vi "IDS_RILIS_V2.vi"() -> ()   [LabVIEW 2015]
uses:
  Case_Selector.ctl
  <vilib>/Utility/file.llb/Read Delimited Spreadsheet (DBL).vi
panel:
  in  "Manual Start":bool
  out "Integral2":dbl
  out "Integral1":dbl
  out "IDS Spectrum":cluster{"all rows":dbl[], "all rows":dbl[]}(graph)
  out "Run Number":dbl
  out "Path":string
  out "IDS_Status.sh - ERROR":string
  out "IDS_Sort.sh - ERROR":string
  out "IDS Data Taking":bool
  out "IDS Sorting":bool
  out "loop counter":i32
  out "RILIS ERROR":bool
  out "IDS ERROR":bool
  out "RILIS Ready":bool
  out "HFS Scan Graph 2":cluster{"Y":dbl[], "Y":dbl[]}[](graph)
  out "Integral":dbl[](array[numeric]) format="%#.2f"
  out "?":string
  out "IDS Ready":bool
  out "IDS_Start.sh - ERROR":string
  out "?":string
  out "Wavenumber Stdev":dbl
  out "Proton Pulses in SC":dbl format="%#_10g"
  out "Full Name":string
  out "created path":path
  in  "stop":bool
  out "Proton Pulse":bool
  out "Super Cycle":bool
  out "protons per pulse":dbl
  out "StepNumber":i32
  out "Wavenumber":dbl format="%#_11g"
  out "Measurement time stamp":timestamp
  out "Laser Power":dbl format="%#_11g"
  out "Integrated current":dbl
  in  "File Base":string
  # "Measurement time stamp"
  # "Output"
  # "RILIS"
  # "Separator"
  # "IDS"
  # "Results"
  # "Last update: 22 May 2022 \nAuthors: Ralf Erik Rossel, Razvan Lica, Rob Harding"
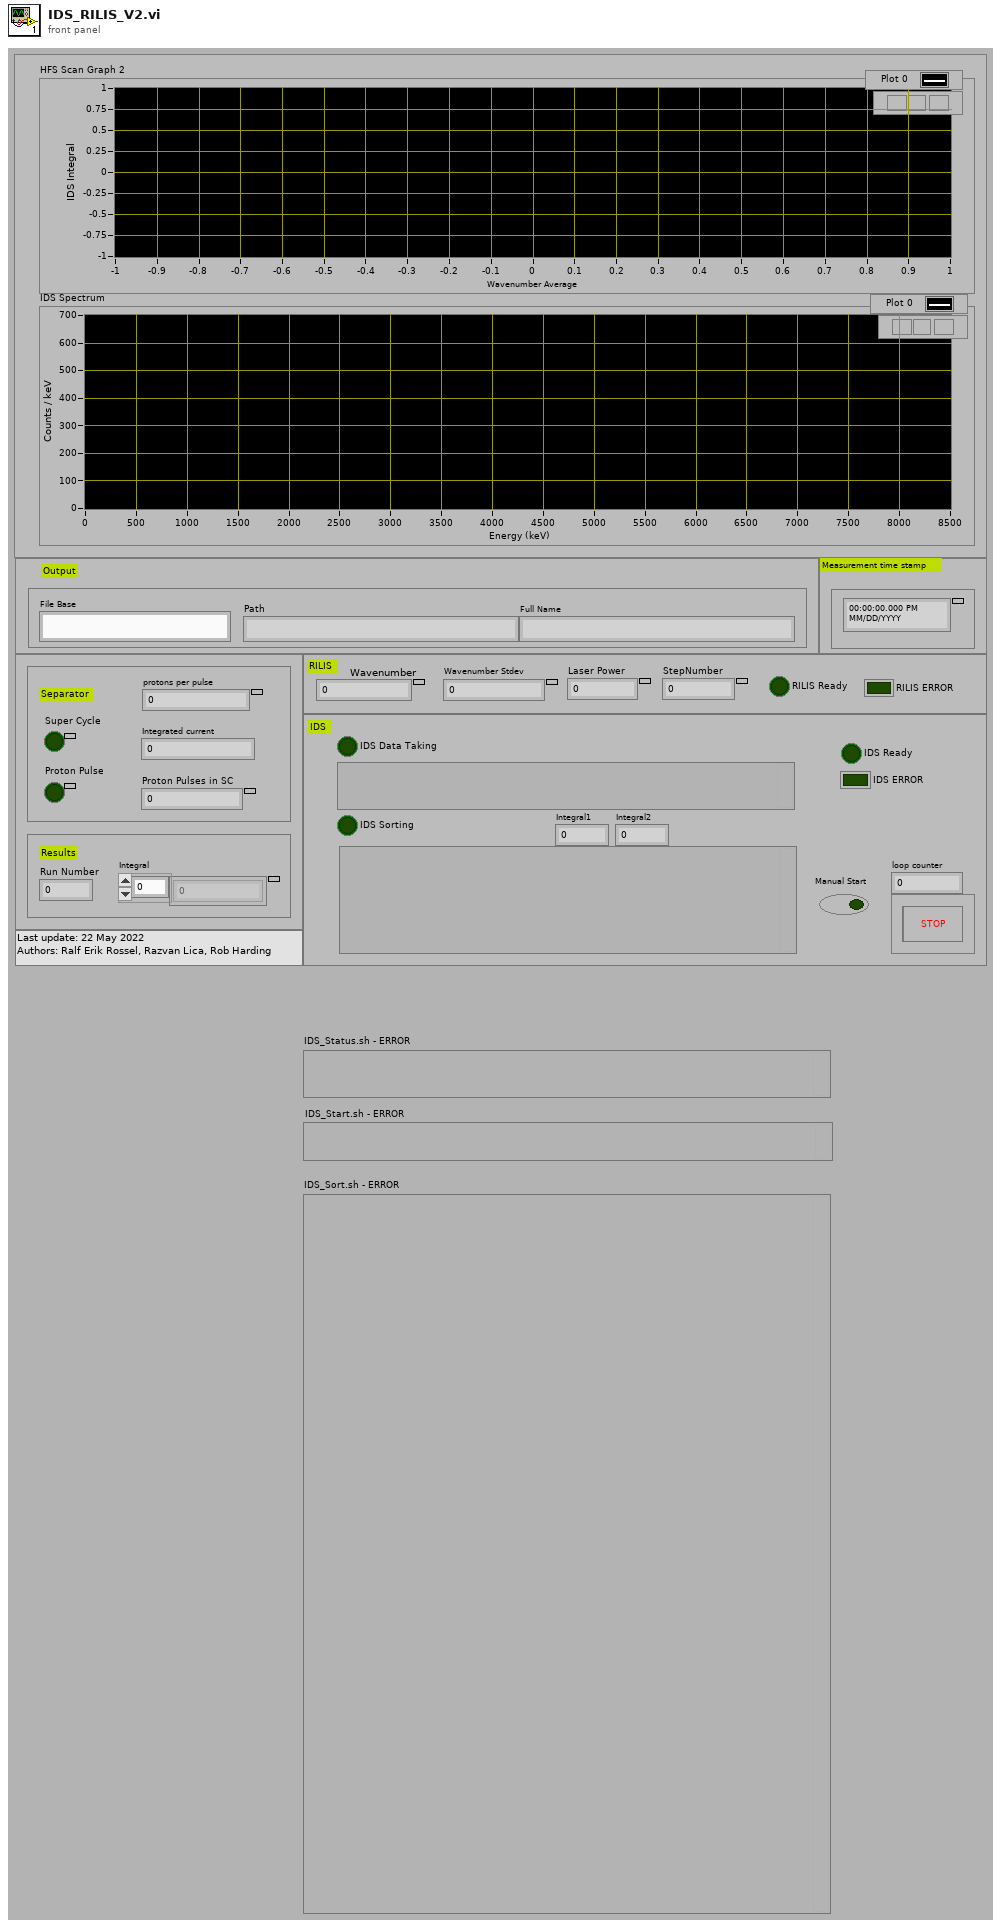
[diagram p1: front panel]
types:
  T1 = typedef "Case_Selector.ctl" = enum16{"RILIS Init", "RILIS On", "RILIS AQN", "RILIS SORT"}
  T2 = enum16{"open", "replace", "create", "open or create", "replace or create", "replace or create with confirmation"}
  T3 = enum16{"Read", "Write", "ReadWrite", "BufferedRead", "BufferedReadWrite"}
  T4 = cluster{"[0]":dbl, "[1]":dbl, "[2]":dbl, "[3]":dbl, "[4]":dbl, "[5]":dbl, "[6]":dbl, "[7]":dbl, "[8]":dbl}
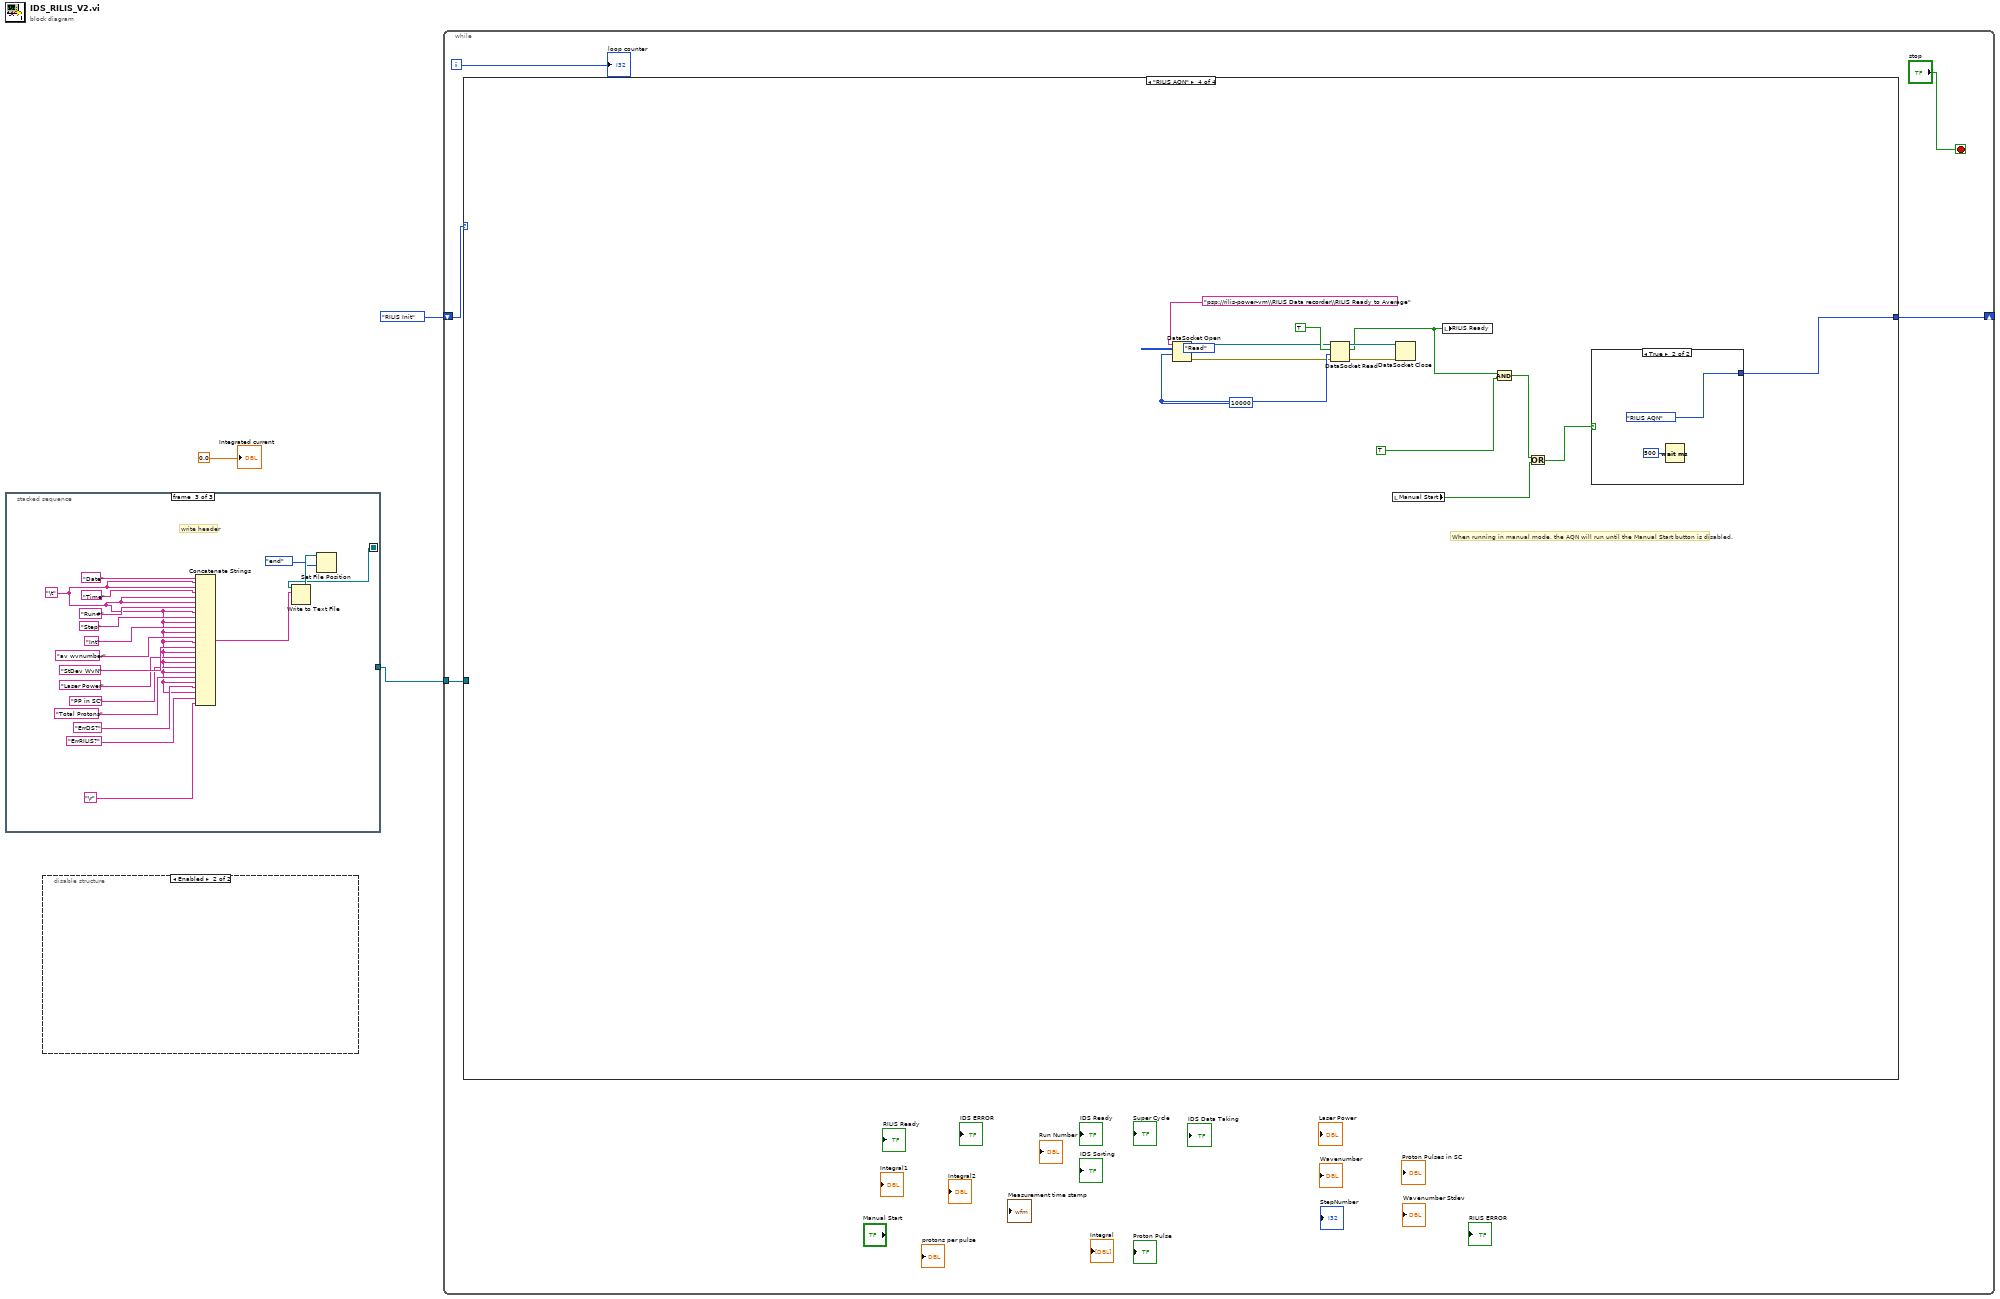
[diagram p0: block diagram]
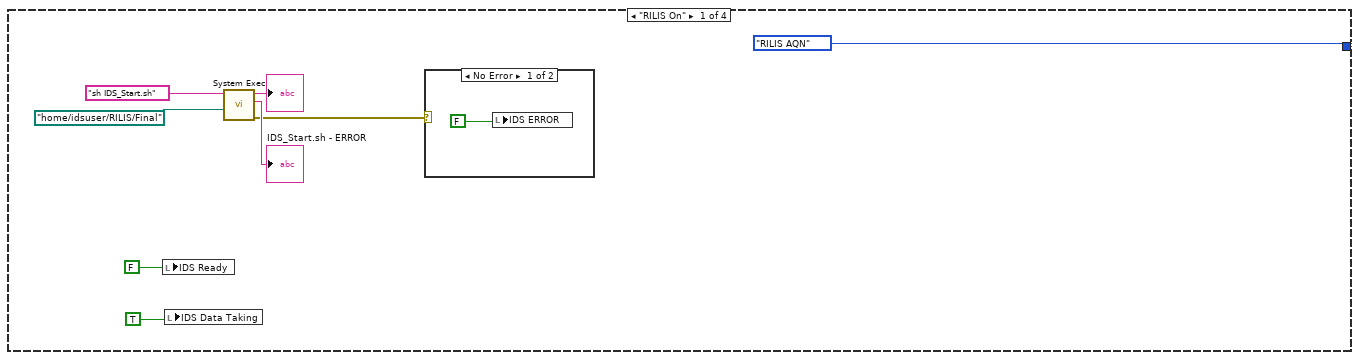
[diagram p2: hidden frame]
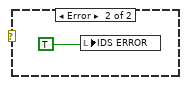
[diagram p3: hidden frame]
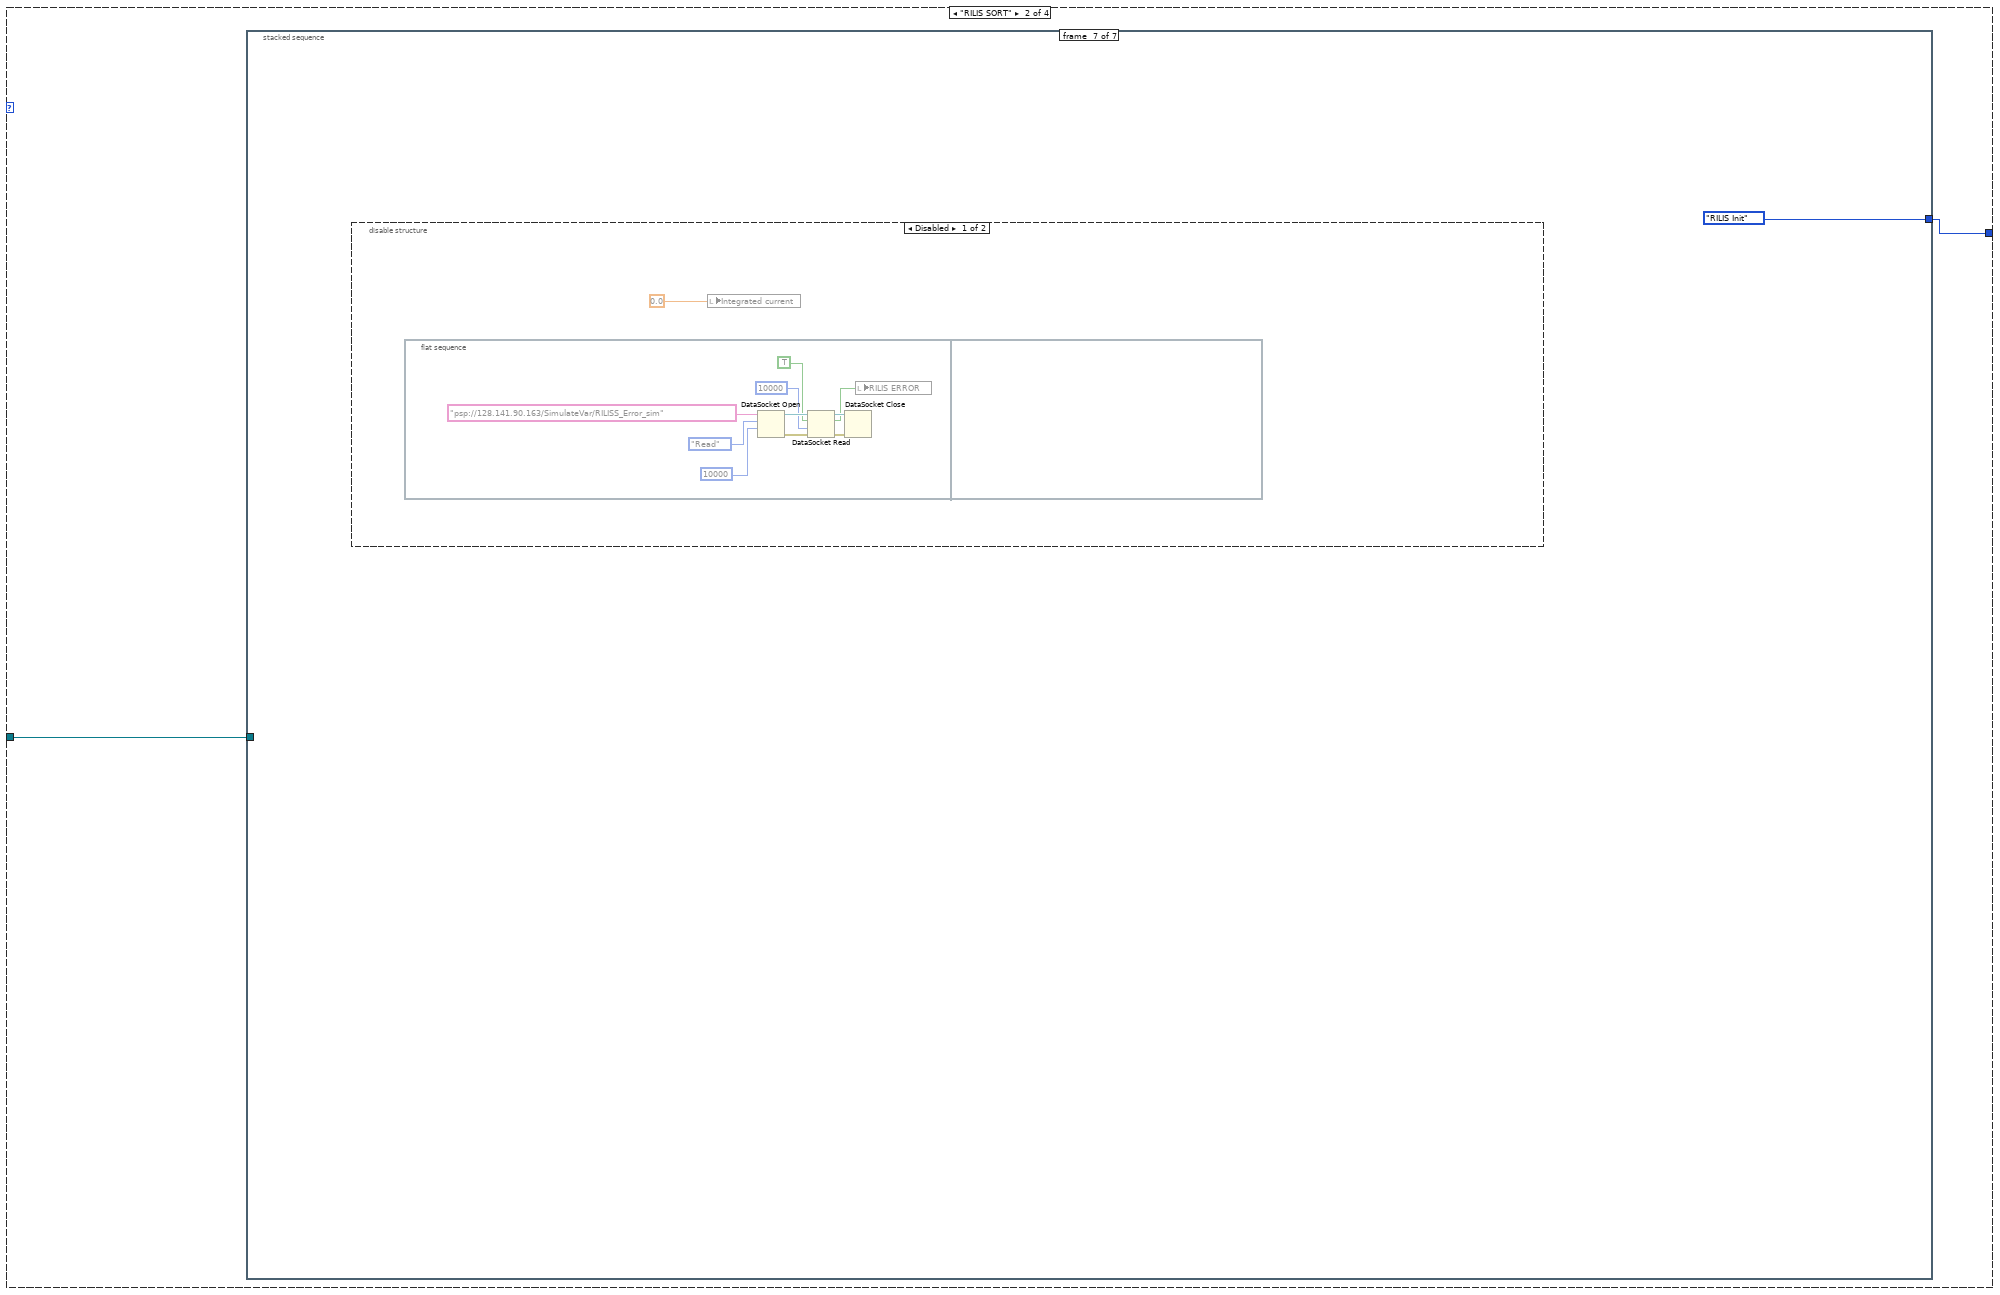
[diagram p4: hidden frame]
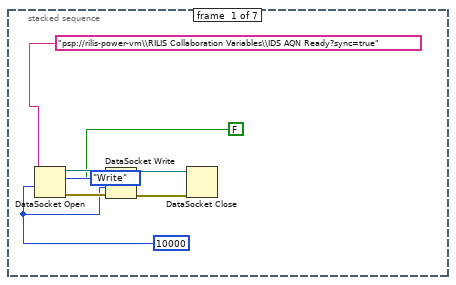
[diagram p5: hidden frame]
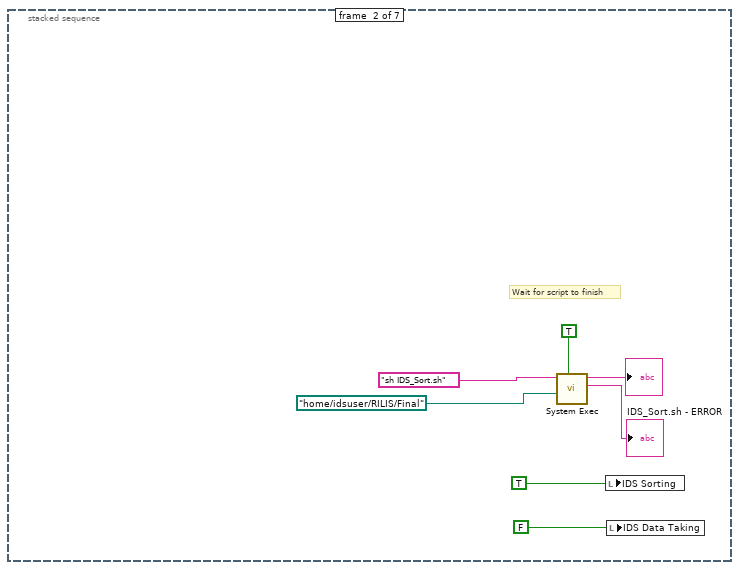
[diagram p6: hidden frame]
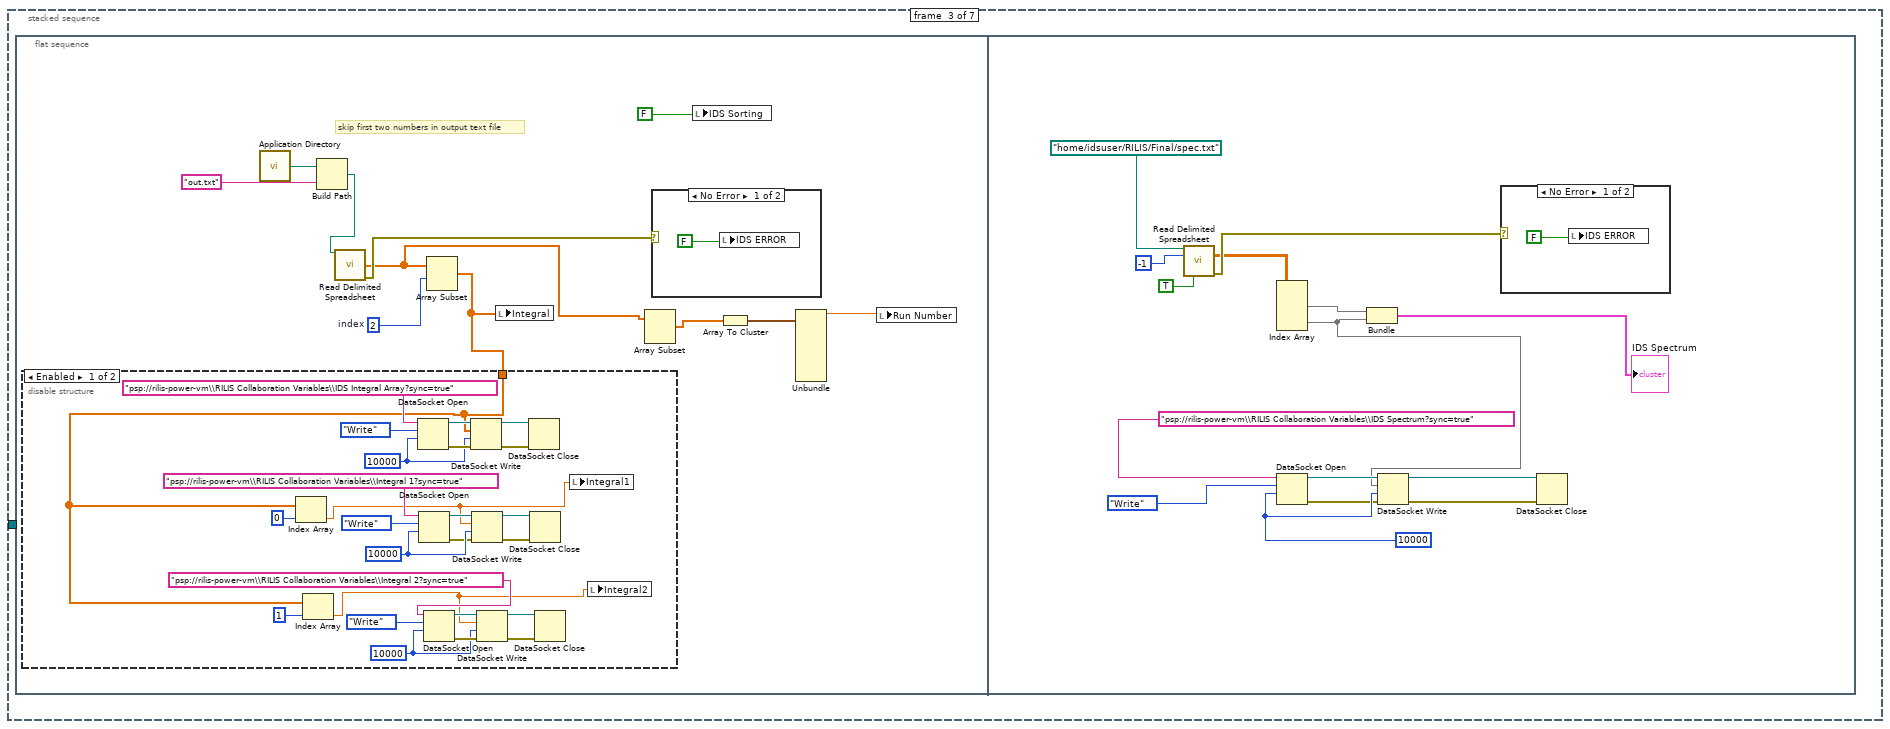
[diagram p7: hidden frame]
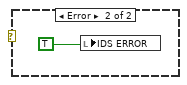
[diagram p9: hidden frame]
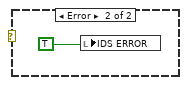
[diagram p10: hidden frame]
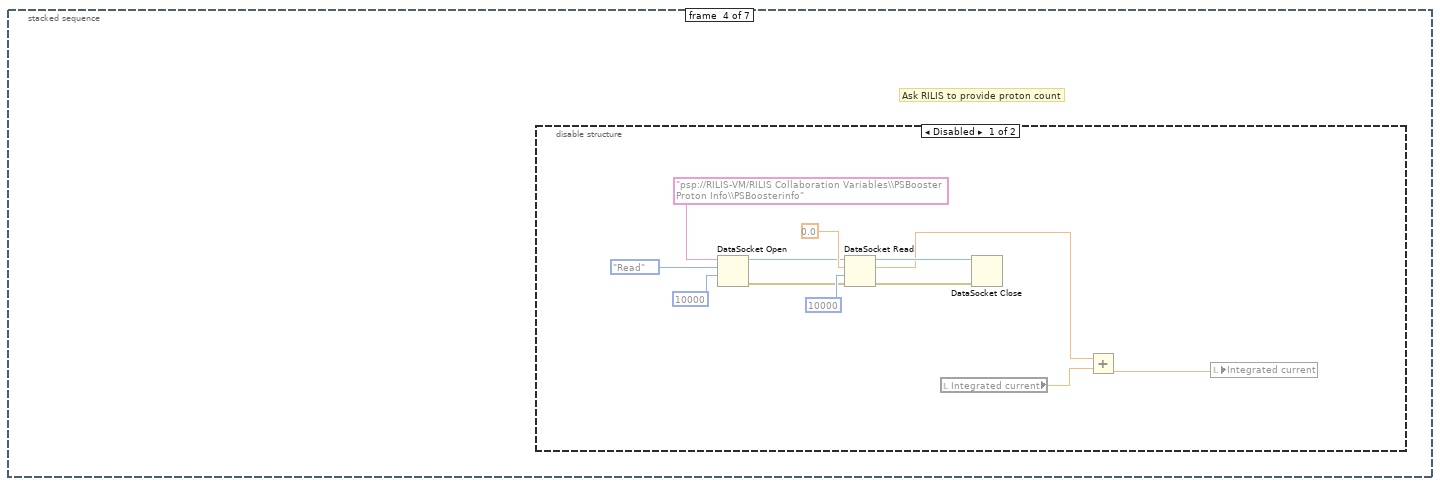
[diagram p11: hidden frame]
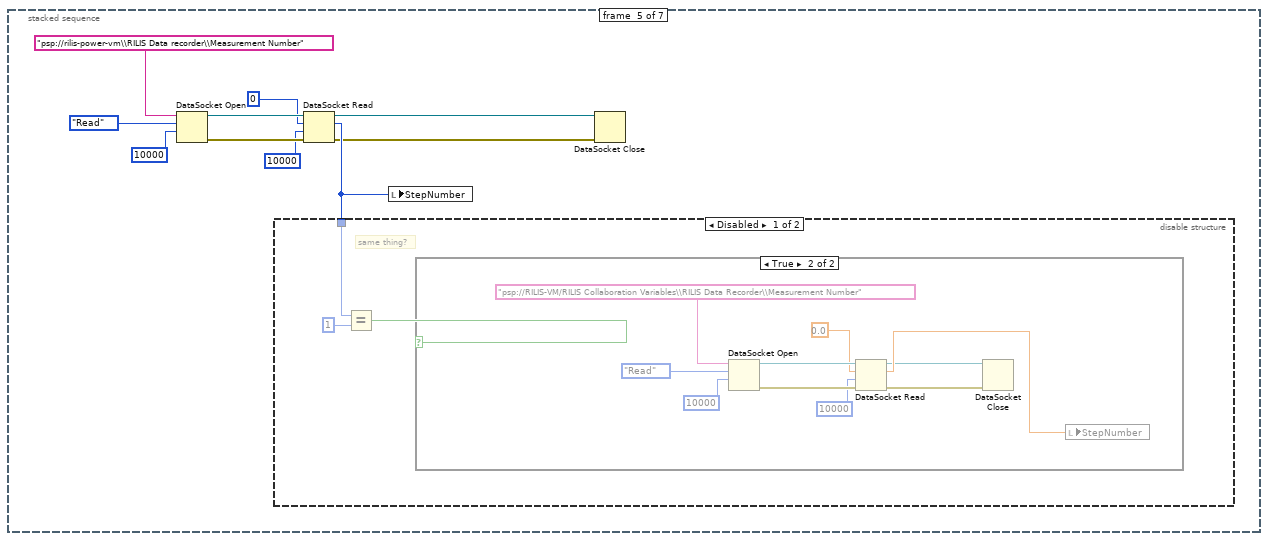
[diagram p13: hidden frame]
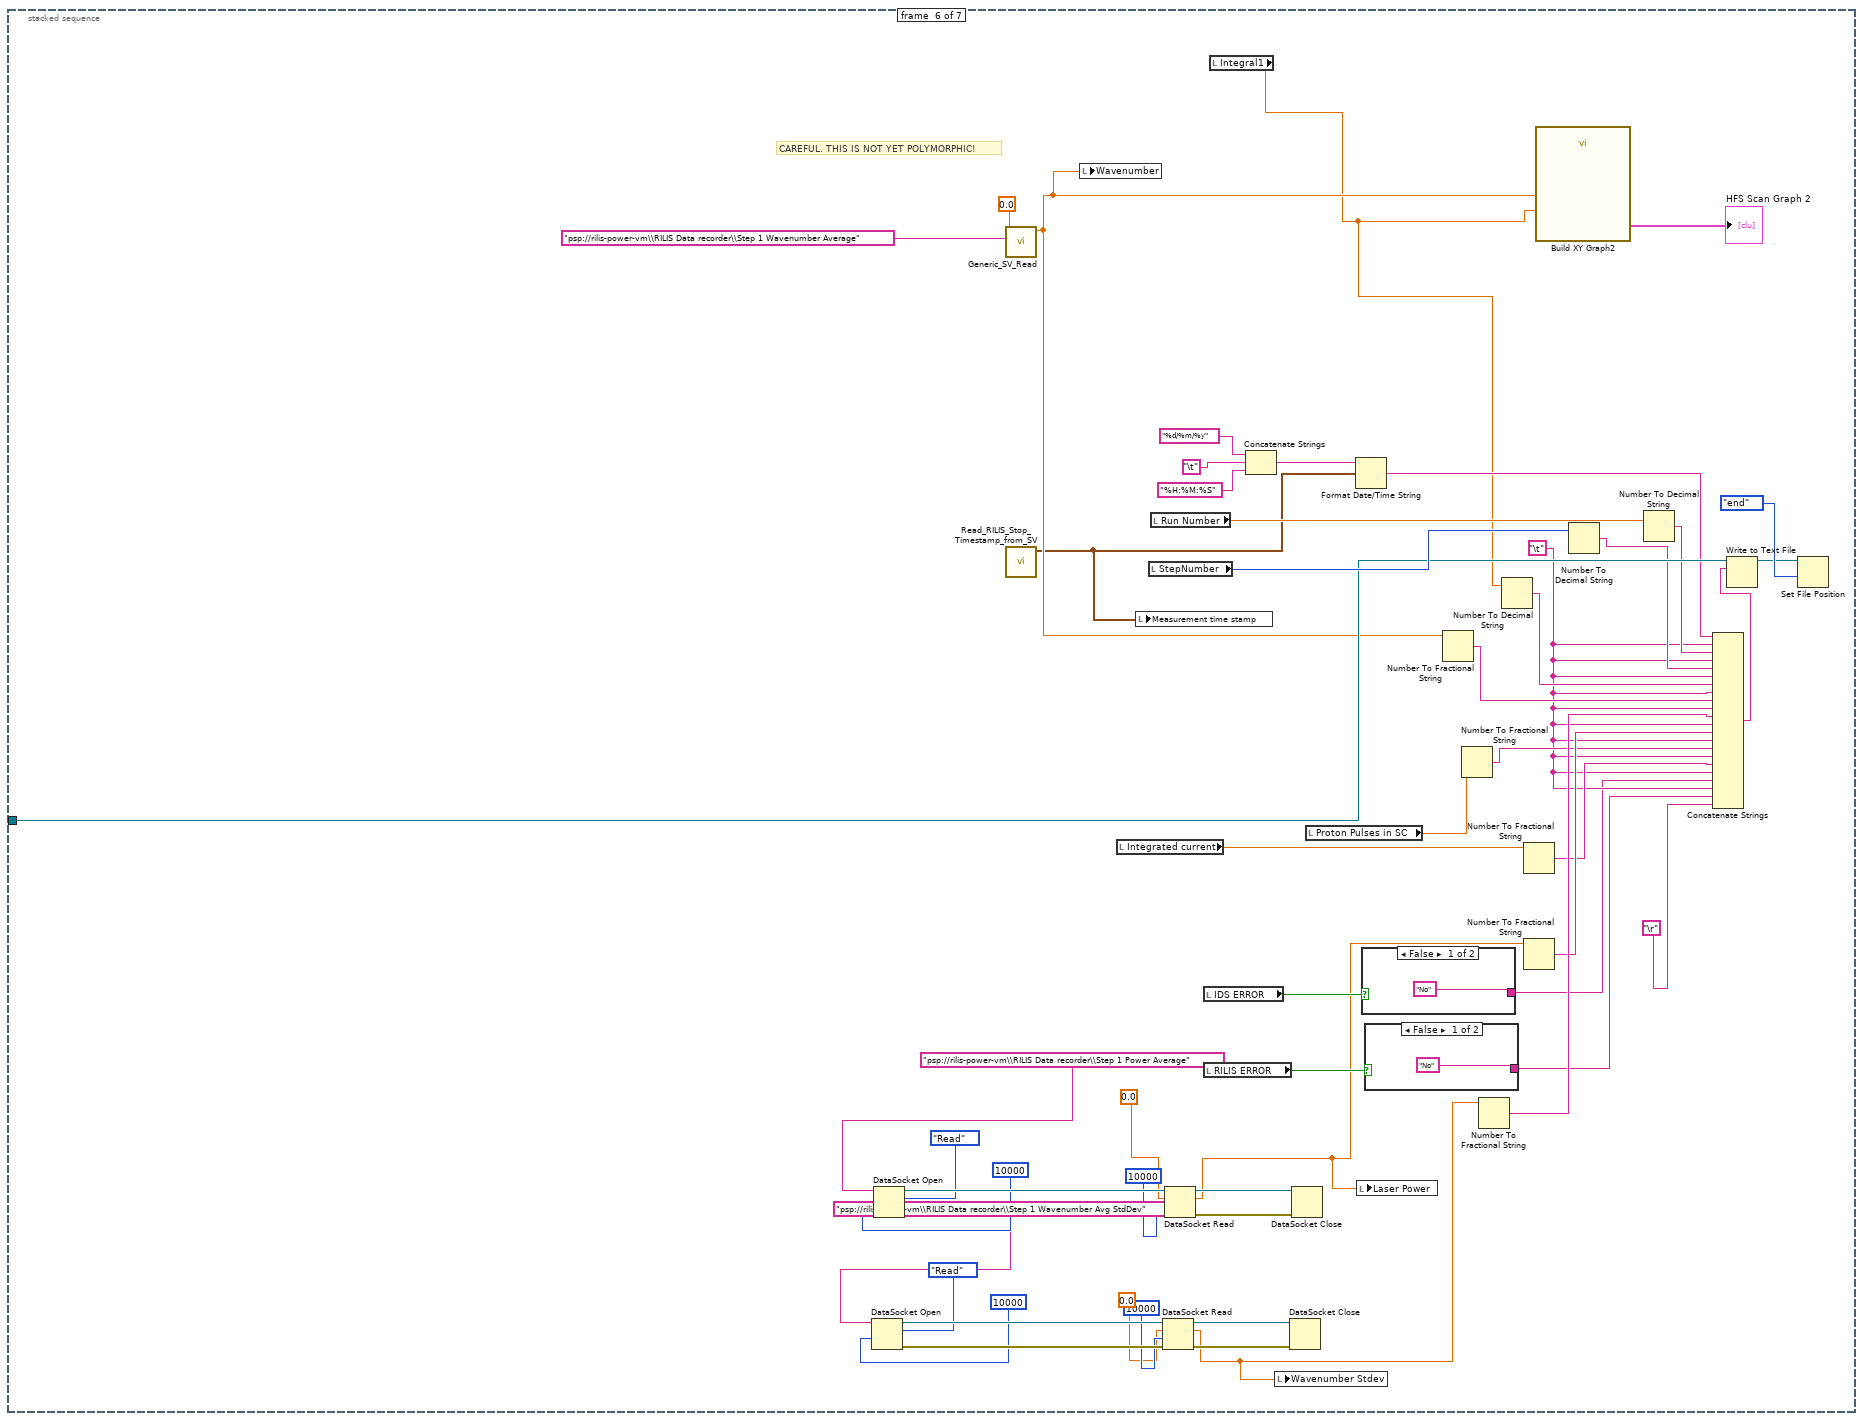
[diagram p16: hidden frame]
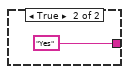
[diagram p17: hidden frame]
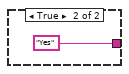
[diagram p18: hidden frame]
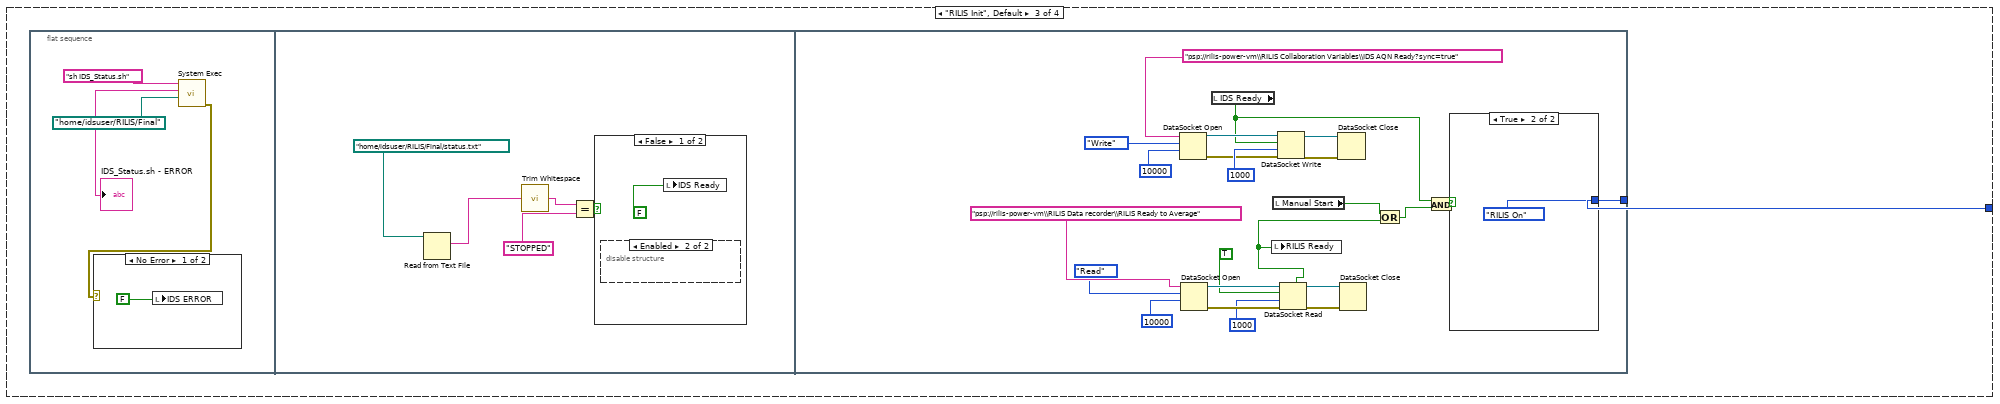
[diagram p20: hidden frame]
diagram:
  n1 = stacked-sequence {
    seq-local: [_ w23 _] -> [_ _ w42]
    tunnel: [_ w23 _] -> w2
    frame #0 {
      w4 = "/home/idsuser/RILIS/"
      w22 = "_"
      w20 = "-" ("replace string (\"\")")
      w19 = "/" ("search string")
      n2 = Get Date/Time String() -> (date string=w17:string, time string=w14:string)  [unwired: 3 in]
      n3 = Search and Replace String(input string=w17, search string=w19, replace string=w20) -> (result string=w18:string)  [unwired: 5 in, 3 out]
      n4 = Search and Replace String(input string=w14, search string=":", replace string="u" ("replace string (\"\")")) -> (result string=w10:string)  [unwired: 5 in, 3 out]
      n5 = String To Path(string=w4) -> (path=w5:path)
      n6 = Search and Replace String(input string=w18, search string=w19, replace string=w20) -> (result string=w9:string)  [unwired: 5 in, 3 out]
      n7 = Search and Replace String(input string=w10, search string=" ", replace string="_" ("replace string (\"\")")) -> (result string=w6:string)  [unwired: 5 in, 3 out]
      n8 = Concatenate Strings(w9, w22, w6, w22, "File Base") -> (w12:string)
      "Full Name" <- w12
      n9 = Build Path(base path=w5, name or relative path=w12) -> (appended path=w13:path)
      n10 = Create Folder(path (use dialog)=w13) -> (created path=→"created path":path)  [unwired: 2 in, 2 out]
      "Path" <- w4
    }
    frame #1 {
      n11 = local read "Full Name"() -> (w24:string)
      n12 = local read "created path"() -> (w25:path)
      n13 = Concatenate Strings(w24, ".txt" ("string")) -> (w27:string)
      n14 = Build Path(base path=w25, name or relative path=w27) -> (appended path=w26:path)
      n15 = Open/Create/Replace File(file path (use dialog)=w26, operation (0:open)=T2."open or create") -> (refnum out=w23:refnum<file>)  [unwired: 4 in, 2 out]
    }
    frame #2 {
      w30 = "\t"
      # "write header"
      n16 = Concatenate Strings("Date" ("string"), w30, w30, "Time" ("string"), w30, w30, "Run#" ("string"), w30, "Step" ("string"), w30, "Int" ("string"), w30, "av wvnumber" ("string"), w30, "StDev WvN" ("string"), w30, "Laser Power" ("string"), w30, "PP in SC" ("string"), w30, "Total Protons" ("string"), w30, "ErrDS?" ("string"), w30, "ErrRILIS?" ("string"), "\r") -> (w43:string)
      n17 = Write to Text File(file (use dialog)=w42, text=w43) -> (refnum out=w47:refnum<file>)  [unwired: 2 in, 2 out]
      n18 = Set File Position(refnum=w47, from (0:start)=enum16{"start", "end", "current"}."end") -> ()  [unwired: 2 in, 2 out]
    }
  }
  n19 = disable-structure shown="Enabled" {
    frame Disabled {
      n20 = flat-sequence {
        frame #0 {
          n21 = DataSocket Open(9:10000 ("ms timeout (10000)"), 10:T3."Read" ("mode"), 11:"psp://128.141.90.163/SimulateVar/RILISS_SS" ("URL")) -> (0:w52:errorcluster, 3:w54:refnum<k13>)  [unwired: 1 in]
          n22 = while {
            tunnel: w54 -> [w61]
            tunnel: [w60] -> w53
            tunnel: w52 -> [w59]
            tunnel: [w56] -> w51
            stop <- w56 stop-if-true
            n23 = DataSocket Read(8:w59, 9:10000 ("ms timeout (10000)"), 10:0.0, 11:w61) -> (0:w56:errorcluster, 2:w57:dbl, 3:w60:refnum<k13>)  [unwired: 1 in, 4 out]
          }
          n24 = DataSocket Close(8:w51, 11:w53) -> ()  [unwired: 1 in, 2 out]
        }
      }
    }
    frame Enabled {
    }
  }
  n25 = while {
    shift-right: [w66] -> _
    shift-left: Case_Selector."RILIS Init" -> [w63]
    tunnel: w2 -> [w65]
    i -> [w64]
    stop <- "stop" stop-if-true
    n26 = case shown="\"RILIS AQN\"" w63 {
      tunnel: [Case_Selector."RILIS AQN" w77 w254 w299] -> w66
      tunnel: w65 -> [_ w78 _ _]
      frame "RILIS On" {
        n27 = local write "IDS Ready"(FALSE) -> ()
        n28 = local write "IDS Data Taking"(TRUE) -> ()
        n29 = call <vilib>:"System Exec.vi"("working directory"=path "/home/idsuser/RILIS/Final", "command line"="sh IDS_Start.sh") -> ("error out"=w67:errorcluster, "standard error"=→"IDS_Start.sh - ERROR":string, "standard output"=→"?":string)  [unwired: 6 in, 1 out]
        n30 = case shown="No Error" w67 {
          frame No Error {
            n31 = local write "IDS ERROR"(FALSE) -> ()
          }
          frame Error {
            n32 = local write "IDS ERROR"(TRUE) -> ()
          }
        }
      }
      frame "RILIS SORT" {
        n33 = stacked-sequence {
          tunnel: w78 -> [_ _ _ _ _ w204 _]
          tunnel: [_ _ _ _ _ _ Case_Selector."RILIS Init"] -> w77
          frame #0 {
            w79 = 10000 ("ms timeout (10000)")
            n34 = DataSocket Open(9:w79, 10:T3."Write" ("mode"), 11:"psp://rilis-power-vm\\RILIS Collaboration Variables\\IDS AQN Ready?sync=true" ("URL")) -> (0:w82:errorcluster, 3:w84:refnum<k13>)  [unwired: 1 in]
            n35 = DataSocket Write(8:w82, 9:w79, 10:FALSE, 11:w84) -> (0:w81:errorcluster, 3:w83:refnum<k13>)  [unwired: 1 out]
            n36 = DataSocket Close(8:w81, 11:w83) -> ()  [unwired: 1 in, 2 out]
          }
          frame #1 {
            # "Wait for script to finish"
            n37 = call <vilib>:"System Exec.vi"("wait until completion? (T)"=TRUE, "working directory"=path "/home/idsuser/RILIS/Final", "command line"="sh IDS_Sort.sh") -> ("standard error"=→"IDS_Sort.sh - ERROR":string, "standard output"=→"?":string)  [unwired: 5 in, 2 out]
            n38 = local write "IDS Sorting"(TRUE) -> ()
            n39 = local write "IDS Data Taking"(FALSE) -> ()
          }
          frame #2 {
            n40 = flat-sequence {
              frame #0 {
                w101 = 2  # index
                # "skip first two numbers in output text file"
                n41 = call <vilib>:"Application Directory.vi"() -> ("Application Directory"=w104:path)
                n42 = Build Path(base path=w104, name or relative path="out.txt") -> (appended path=w103:path)
                n43 = call-poly <vilib>:"Read Delimited Spreadsheet.vi"("file path (dialog if empty)"=w103) -> ("first row"=w95:dbl[], "error out"=w99:errorcluster)  [unwired: 9 in, 4 out]
                n44 = Array Subset(array=w95, index=w101) -> (w94:dbl[])  [unwired: 1 in]
                n45 = disable-structure shown="Enabled" {
                  disable-tunnel: w94 -> [w108 _]
                  frame Enabled {
                    w111 = 10000 ("ms timeout (10000)")
                    w122 = 10000 ("ms timeout (10000)")
                    w125 = 10000 ("ms timeout (10000)")
                    n46 = Index Array(array=w108, index=0) -> (element=w106:dbl)
                    n47 = Index Array(array=w108, index=1) -> (element=w105:dbl)
                    n48 = DataSocket Open(9:w125, 10:T3."Write" ("mode"), 11:"psp://rilis-power-vm\\RILIS Collaboration Variables\\IDS Integral Array?sync=true" ("URL")) -> (0:w128:errorcluster, 3:w129:refnum<k13>)  [unwired: 1 in]
                    n49 = DataSocket Open(9:w122, 10:T3."Write" ("mode"), 11:"psp://rilis-power-vm\\RILIS Collaboration Variables\\Integral 1?sync=true" ("URL")) -> (0:w119:errorcluster, 3:w118:refnum<k13>)  [unwired: 1 in]
                    n50 = DataSocket Open(9:w111, 10:T3."Write" ("mode"), 11:"psp://rilis-power-vm\\RILIS Collaboration Variables\\Integral 2?sync=true" ("URL")) -> (0:w114:errorcluster, 3:w115:refnum<k13>)  [unwired: 1 in]
                    n51 = DataSocket Write(8:w128, 9:w125, 10:w108, 11:w129) -> (0:w127:errorcluster, 3:w126:refnum<k13>)  [unwired: 1 out]
                    n52 = DataSocket Write(8:w119, 9:w122, 10:w106, 11:w118) -> (0:w120:errorcluster, 3:w121:refnum<k13>)  [unwired: 1 out]
                    n53 = DataSocket Write(8:w114, 9:w111, 10:w105, 11:w115) -> (0:w113:errorcluster, 3:w112:refnum<k13>)  [unwired: 1 out]
                    n54 = DataSocket Close(8:w127, 11:w126) -> ()  [unwired: 1 in, 2 out]
                    n55 = DataSocket Close(8:w120, 11:w121) -> ()  [unwired: 1 in, 2 out]
                    n56 = DataSocket Close(8:w113, 11:w112) -> ()  [unwired: 1 in, 2 out]
                    n57 = local write "Integral1"(w106) -> ()
                    n58 = local write "Integral2"(w105) -> ()
                  }
                  frame Disabled {
                  }
                }
                n59 = local write "Integral"(w94) -> ()
                n60 = Array Subset(array=w95) -> (w97:dbl[])  [unwired: 2 in]
                n61 = case shown="No Error" w99 {
                  frame No Error {
                    n62 = local write "IDS ERROR"(FALSE) -> ()
                  }
                  frame Error {
                    n63 = local write "IDS ERROR"(TRUE) -> ()
                  }
                }
                n64 = local write "IDS Sorting"(FALSE) -> ()
                n65 = Array To Cluster(array=w97) -> (cluster=w98:T4)
                n66 = Unbundle(w98) -> ("[0]"=w96:dbl)  [unwired: 8 out]
                n67 = local write "Run Number"(w96) -> ()
              }
              frame #1 {
                w145 = 10000 ("ms timeout (10000)")
                n68 = call-poly <vilib>:"Read Delimited Spreadsheet.vi"("file path (dialog if empty)"=path "/home/idsuser/RILIS/Final/spec.txt", "number of rows (all:-1)"=-1, "transpose? (F)"=TRUE) -> ("all rows"=w139:dbl[][], "error out"=w147:errorcluster)  [unwired: 7 in, 4 out]
                n69 = Index Array(array=w139) -> (element #1=w138:dbl[], element #2=w137:dbl[])  [unwired: 4 in]
                n70 = DataSocket Open(9:w145, 10:T3."Write" ("mode"), 11:"psp://rilis-power-vm\\RILIS Collaboration Variables\\IDS Spectrum?sync=true" ("URL")) -> (0:w142:errorcluster, 3:w141:refnum<k13>)  [unwired: 1 in]
                n71 = Bundle("all rows"=w138, "all rows"=w137) -> (→"IDS Spectrum":cluster{"all rows":dbl[], "all rows":dbl[]})  [unwired: 1 in]
                n72 = DataSocket Write(8:w142, 9:w145, 10:w137, 11:w141) -> (0:w143:errorcluster, 3:w144:refnum<k13>)  [unwired: 1 out]
                n73 = case shown="No Error" w147 {
                  frame No Error {
                    n74 = local write "IDS ERROR"(FALSE) -> ()
                  }
                  frame Error {
                    n75 = local write "IDS ERROR"(TRUE) -> ()
                  }
                }
                n76 = DataSocket Close(8:w143, 11:w144) -> ()  [unwired: 1 in, 2 out]
              }
            }
          }
          frame #3 {
            # "Ask RILIS to provide proton count"
            n77 = disable-structure shown="Disabled" {
              frame Disabled {
                n78 = DataSocket Open(9:10000 ("ms timeout (10000)"), 10:T3."Read" ("mode"), 11:"psp://RILIS-VM/RILIS Collaboration Variables\\PSBooster Proton Info\\PSBoosterinfo" ("URL")) -> (0:w154:errorcluster, 3:w153:refnum<k13>)  [unwired: 1 in]
                n79 = DataSocket Read(8:w154, 9:10000 ("ms timeout (10000)"), 10:0.0, 11:w153) -> (0:w161:errorcluster, 2:w150:dbl, 3:w158:refnum<k13>)  [unwired: 1 in, 4 out]
                n80 = local read "Integrated current"() -> (w152:dbl)
                n81 = DataSocket Close(8:w161, 11:w158) -> ()  [unwired: 1 in, 2 out]
                n82 = Add(x=w150, y=w152) -> (x+y=w151:dbl)
                n83 = local write "Integrated current"(w151) -> ()
              }
              frame Enabled {
              }
            }
          }
          frame #4 {
            n84 = DataSocket Open(9:10000 ("ms timeout (10000)"), 10:T3."Read" ("mode"), 11:"psp://rilis-power-vm\\RILIS Data recorder\\Measurement Number" ("URL")) -> (0:w169:errorcluster, 3:w170:refnum<k13>)  [unwired: 1 in]
            n85 = DataSocket Read(8:w169, 9:10000 ("ms timeout (10000)"), 10:0, 11:w170) -> (0:w162:errorcluster, 2:w171:i32, 3:w165:refnum<k13>)  [unwired: 1 in, 4 out]
            n86 = disable-structure shown="Disabled" {
              disable-tunnel: w171 -> [w174 _]
              frame Disabled {
                # "same thing?"
                n87 = Equal?(x=w174, y=1) -> (x = y?=w173:bool)
                n88 = case shown="True" w173 {
                  frame False {
                  }
                  frame True {
                    n89 = DataSocket Open(9:10000 ("ms timeout (10000)"), 10:T3."Read" ("mode"), 11:"psp://RILIS-VM/RILIS Collaboration Variables\\RILIS Data Recorder\\Measurement Number" ("URL")) -> (0:w182:errorcluster, 3:w183:refnum<k13>)  [unwired: 1 in]
                    n90 = DataSocket Read(8:w182, 9:10000 ("ms timeout (10000)"), 10:0.0, 11:w183) -> (0:w175:errorcluster, 2:w184:dbl, 3:w178:refnum<k13>)  [unwired: 1 in, 4 out]
                    n91 = DataSocket Close(8:w175, 11:w178) -> ()  [unwired: 1 in, 2 out]
                    n92 = local write "StepNumber"(w184) -> ()
                  }
                }
              }
              frame Enabled {
              }
            }
            n93 = local write "StepNumber"(w171) -> ()
            n94 = DataSocket Close(8:w162, 11:w165) -> ()  [unwired: 1 in, 2 out]
          }
          frame #5 {
            w190 = "\t"
            # "CAREFUL. THIS IS NOT YET POLYMORPHIC!"
            n95 = DataSocket Open(9:10000 ("ms timeout (10000)"), 10:T3."Read" ("mode"), 11:"psp://rilis-power-vm\\RILIS Data recorder\\Step 1 Wavenumber Avg StdDev" ("URL")) -> (0:w214:errorcluster, 3:w215:refnum<k13>)  [unwired: 1 in]
            n96 = DataSocket Open(9:10000 ("ms timeout (10000)"), 10:T3."Read" ("mode"), 11:"psp://rilis-power-vm\\RILIS Data recorder\\Step 1 Power Average" ("URL")) -> (0:w221:errorcluster, 3:w222:refnum<k13>)  [unwired: 1 in]
            n97 = call "Generic_SV_Read.vi"("SV URL"="psp://rilis-power-vm\\RILIS Data recorder\\Step 1 Wavenumber Average" ("URL"), "type in"=0.0) -> ("Data out"=w203:dbl)  [unwired: 9 in]
            n98 = call "Read_RILIS_Stop_Timestamp_from_SV.vi"() -> ("Time Stamp"=w186:timestamp)  [unwired: 11 in]
            n99 = local write "Wavenumber"(w203) -> ()
            n100 = local read "Integrated current"() -> (w232:dbl)
            n101 = local write "Measurement time stamp"(w186) -> ()
            n102 = local read "StepNumber"() -> (w236:i32)
            n103 = local read "Run Number"() -> (w199:dbl)
            n104 = DataSocket Read(8:w214, 9:10000 ("ms timeout (10000)"), 10:0.0, 11:w215) -> (0:w213:errorcluster, 2:w201:dbl, 3:w209:refnum<k13>)  [unwired: 1 in, 4 out]
            n105 = DataSocket Read(8:w221, 9:10000 ("ms timeout (10000)"), 10:0.0, 11:w222) -> (0:w220:errorcluster, 2:w202:dbl, 3:w216:refnum<k13>)  [unwired: 1 in, 4 out]
            n106 = local read "IDS ERROR"() -> (w234:bool)
            n107 = local read "RILIS ERROR"() -> (w235:bool)
            n108 = local read "Integral1"() -> (w185:dbl)
            n109 = Concatenate Strings("%d/%m/%y" ("time format string (%c)"), "\t", "%H:%M:%S" ("time format string (%c)")) -> (w229:string)
            n110 = local write "Wavenumber Stdev"(w201) -> ()
            n111 = DataSocket Close(8:w213, 11:w209) -> ()  [unwired: 1 in, 2 out]
            n112 = DataSocket Close(8:w220, 11:w216) -> ()  [unwired: 1 in, 2 out]
            n113 = local read "Proton Pulses in SC"() -> (w233:dbl)
            n114 = Format Date/Time String(time format string (%c)=w229, seconds (now)=w186) -> (date/time string=w200:string)  [unwired: 1 in]
            n115 = local write "Laser Power"(w202) -> ()
            n116 = case shown="False" w234 {
              tunnel: ["No" ("string") "Yes" ("string")] -> w189
              frame False {
              }
              frame True {
              }
            }
            n117 = case shown="False" w235 {
              tunnel: ["No" ("string") "Yes" ("string")] -> w188
              frame False {
              }
              frame True {
              }
            }
            n118 = Number To Fractional String(number=w203) -> (F-format string=w195:string)  [unwired: 3 in]
            n119 = Number To Fractional String(number=w233) -> (F-format string=w192:string)  [unwired: 3 in]
            n120 = Number To Fractional String(number=w201) -> (F-format string=w194:string)  [unwired: 3 in]
            n121 = Number To Decimal String(number=w185) -> (decimal integer string=w196:string)  [unwired: 1 in]
            n122 = Number To Fractional String(number=w232) -> (F-format string=w191:string)  [unwired: 3 in]
            n123 = Number To Fractional String(number=w202) -> (F-format string=w193:string)  [unwired: 3 in]
            n124 = call "Build XY Graph2"("Y Input"=w185, "X Input"=w203) -> ("XY Graph"=→"HFS Scan Graph 2":cluster{"Y":dbl[], "Y":dbl[]}[])  [unwired: 8 in, 1 out]
            n125 = Number To Decimal String(number=w236) -> (decimal integer string=w197:string)  [unwired: 1 in]
            n126 = Number To Decimal String(number=w199) -> (decimal integer string=w198:string)  [unwired: 1 in]
            n127 = Concatenate Strings(w200, w190, w198, w190, w197, w190, w196, w190, w195, w190, w194, w190, w193, w190, w192, w190, w191, w190, w189, w190, w188, "\r") -> (w226:string)
            n128 = Write to Text File(file (use dialog)=w204, text=w226) -> (refnum out=w225:refnum<file>)  [unwired: 2 in, 2 out]
            n129 = Set File Position(refnum=w225, from (0:start)=enum16{"start", "end", "current"}."end") -> ()  [unwired: 2 in, 2 out]
          }
          frame #6 {
            n130 = disable-structure shown="Disabled" {
              frame Disabled {
                n131 = flat-sequence {
                  frame #0 {
                    n132 = DataSocket Open(9:10000 ("ms timeout (10000)"), 10:T3."Read" ("mode"), 11:"psp://128.141.90.163/SimulateVar/RILISS_Error_sim" ("URL")) -> (0:w252:errorcluster, 3:w253:refnum<k13>)  [unwired: 1 in]
                    n133 = DataSocket Read(8:w252, 9:10000 ("ms timeout (10000)"), 10:TRUE, 11:w253) -> (0:w251:errorcluster, 2:w244:bool, 3:w247:refnum<k13>)  [unwired: 1 in, 4 out]
                    n134 = DataSocket Close(8:w251, 11:w247) -> ()  [unwired: 1 in, 2 out]
                    n135 = local write "RILIS ERROR"(w244) -> ()
                  }
                  frame #1 {
                  }
                }
                n136 = local write "Integrated current"(0.0 ("Integrated proton current")) -> ()
              }
              frame Enabled {
              }
            }
          }
        }
      }
      frame "RILIS Init", Default {
        n137 = flat-sequence {
          tunnel: [w272] -> w254
          frame #0 {
            n138 = call <vilib>:"System Exec.vi"("working directory"=path "/home/idsuser/RILIS/Final", "command line"="sh IDS_Status.sh") -> ("error out"=w255:errorcluster, "standard error"=→"IDS_Status.sh - ERROR":string)  [unwired: 6 in, 2 out]
            n139 = case shown="No Error" w255 {
              frame No Error {
                n140 = local write "IDS ERROR"(FALSE) -> ()
              }
              frame Error {
                n141 = local write "IDS ERROR"(TRUE) -> ()
              }
            }
          }
          frame #1 {
            n142 = Read from Text File(file (use dialog)=path "/home/idsuser/RILIS/Final/status.txt" ("file path (dialog if empty)")) -> (text=w261:string)  [unwired: 3 in, 3 out]
            n143 = call <vilib>:"Trim Whitespace.vi"("string"=w261) -> ("trimmed string"=w263:string)  [unwired: 1 in]
            n144 = Equal?(x=w263, y="STOPPED") -> (x = y?=w264:bool)
            n145 = case shown="False" w264 {
              frame False {
                n146 = disable-structure shown="Enabled" {
                  frame Disabled {
                    n147 = local write "IDS ERROR"(TRUE) -> ()
                  }
                  frame Enabled {
                  }
                }
                n148 = local write "IDS Ready"(FALSE) -> ()
              }
              frame True {
                n149 = local write "IDS Ready"(TRUE) -> ()
              }
            }
          }
          frame #2 {
            n150 = DataSocket Open(9:10000 ("ms timeout (10000)"), 10:T3."Write" ("mode"), 11:"psp://rilis-power-vm\\RILIS Collaboration Variables\\IDS AQN Ready?sync=true" ("URL")) -> (0:w289:errorcluster, 3:w287:refnum<k13>)  [unwired: 1 in]
            n151 = DataSocket Open(9:10000 ("ms timeout (10000)"), 10:T3."Read" ("mode"), 11:"psp://rilis-power-vm\\RILIS Data recorder\\RILIS Ready to Average" ("URL")) -> (0:w280:errorcluster, 3:w282:refnum<k13>)  [unwired: 1 in]
            n152 = local read "IDS Ready"() -> (w274:bool)
            n153 = local read "Manual Start"() -> (w269:bool)
            n154 = DataSocket Write(8:w289, 9:1000 ("ms timeout (0)"), 10:w274, 11:w287) -> (0:w290:errorcluster, 3:w288:refnum<k13>)  [unwired: 1 out]
            n155 = DataSocket Read(8:w280, 9:1000 ("ms timeout (0)"), 10:TRUE, 11:w282) -> (0:w279:errorcluster, 2:w271:bool, 3:w281:refnum<k13>)  [unwired: 1 in, 4 out]
            n156 = local write "RILIS Ready"(w271) -> ()
            n157 = DataSocket Close(8:w290, 11:w288) -> ()  [unwired: 1 in, 2 out]
            n158 = DataSocket Close(8:w279, 11:w281) -> ()  [unwired: 1 in, 2 out]
            n159 = Or(x=w269, y=w271) -> (x .or. y?=w270:bool)
            n160 = And(x=w274, y=w270) -> (x .and. y?=w273:bool)
            n161 = case shown="True" w273 {
              tunnel: [Case_Selector."RILIS Init" Case_Selector."RILIS On"] -> w272
              frame False {
                # "wait for 50 ms\nto ask rilis again\nfor status"
                n162 = Wait (ms)(milliseconds to wait=u32 50) -> ()  [unwired: 1 out]
              }
              frame True {
              }
            }
          }
        }
      }
      frame "RILIS AQN" {
        w307 = 10000 ("ms timeout (10000)")
        # "When running in manual mode, the AQN will run until the Manual Start button is disabled."
        n163 = DataSocket Open(9:w307, 10:T3."Read" ("mode"), 11:"psp://rilis-power-vm\\RILIS Data recorder\\RILIS Ready to Average" ("URL")) -> (0:w305:errorcluster, 3:w304:refnum<k13>)  [unwired: 1 in]
        n164 = DataSocket Read(8:w305, 9:w307, 10:TRUE, 11:w304) -> (0:w303:errorcluster, 2:w301:bool, 3:w302:refnum<k13>)  [unwired: 1 in, 4 out]
        n165 = local read "Manual Start"() -> (w295:bool)
        n166 = DataSocket Close(8:w303, 11:w302) -> ()  [unwired: 1 in, 2 out]
        n167 = local write "RILIS Ready"(w301) -> ()
        n168 = And(x=w301, y=TRUE) -> (x .and. y?=w297:bool)
        n169 = Or(x=w297, y=w295) -> (x .or. y?=w296:bool)
        n170 = case shown="True" w296 {
          tunnel: [Case_Selector."RILIS SORT" Case_Selector."RILIS AQN"] -> w299
          frame False {
          }
          frame True {
            n171 = Wait (ms)(milliseconds to wait=u32 500) -> ()  [unwired: 1 out]
          }
        }
      }
    }
    "loop counter" <- w64
  }
  "Integrated current" <- 0.0 ("Integrated proton current")
